vi "Initialize.vi"(8 "error in (no error)":errorcluster, 9 "Baudrate":u32, 10 "COM Port":refnum<visa-resource-name>, 11 "Communication in":refnum<class "Communication.lvclass">) -> (0 "error out":errorcluster, 3 "Communication out":refnum<class "Communication.lvclass">)   [LabVIEW 2019, in "Communication.lvclass"]
uses:
  Communication.lvclass
  Communication.lvclass/Communication.ctl
  <vilib>/Instr/_visa.llb/VISA Configure Serial Port (Instr).vi
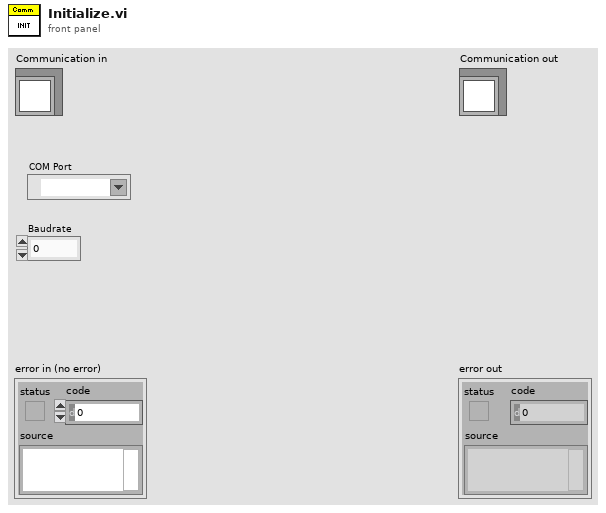
[diagram p1: front panel]
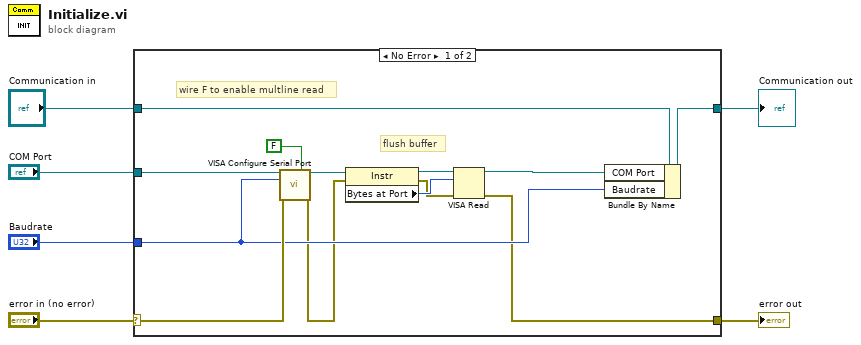
[diagram p0: block diagram]
diagram:
  n1 = case shown="No Error" "error in (no error)" {
    selector: "error in (no error)" -> [w17 w21]
    tunnel: [w7 w21] -> w5
    tunnel: [w18 w20] -> w3
    tunnel: "Communication in" -> [w19 w20]
    tunnel: "Baudrate" -> [w15 _]
    tunnel: "COM Port" -> [w16 _]
    frame No Error {
      # "flush buffer"
      # "wire F to enable multline read"
      n2 = call-poly "VISA Configure Serial Port"("VISA resource name"=w16, "Enable Termination\nChar (T)"=FALSE ("Enable Termination\nChar (T)"), "baud rate (9600)"=w15, "error in (no error)"=w17) -> ("VISA resource name out"=w12:refnum<visa-resource-name>, "error out"=w9:errorcluster)  [unwired: 10 in]
      n3 = property class="Instr"(reference=w12, error in=w9) -> (reference out=w11:refnum<visa-resource-name>, error out=w8:errorcluster, "Bytes at Port"=w13:u32)
      n4 = VISA Read(VISA resource name=w11, byte count=w13, error in (no error)=w8) -> (VISA resource name out=w10:refnum<visa-resource-name>, error out=w7:errorcluster)  [unwired: 2 out]
      n5 = Bundle By Name(cluster=w19, "COM Port"=w10, "Baudrate"=w15) -> (w18:refnum<class "Communication.lvclass">)
    }
    frame Error {
    }
  }
  "error out" <- w5
  "Communication out" <- w3
